vi "Set Toolbar Images.vi"(8 "error in (no error)":errorcluster, 10 "State":T3={"Buttons Displayed"=0, "Button States"=[], "Button Size"=0, "Button Style"=enum."Classic", "Active Button"=0, "Force Regen?"=FALSE, "Tip String Ref"=refnum}) -> (0 "error out":errorcluster, 2 "State Out":T3={"Buttons Displayed"=0, "Button States"=[], "Button Size"=0, "Button Style"=enum."Classic", "Active Button"=0, "Force Regen?"=FALSE, "Tip String Ref"=refnum} caption="State", 3 "Cancelled?":bool)   [LabVIEW 2018, in "Toolbar.xctl"]
doc: "Dialog box to edit the buttons on the toolbar at edit time"
uses:
  Toolbar.xctl
  <vilib>/picture/picture.llb/imagedata.ctl
  Button_Class/Button.lvclass
  Button_Class/Type Defs/Button Status.ctl
  Toolbar State.ctl
  Button_Class/Type Defs/Button Style.ctl
  Button_Class/Type Defs/Button Type.ctl
panel:
  in  "Same Image for all buttons":bool
  out "working Button":refnum<class "Button.lvclass">
  out "Button Images":T1[](array[typedef])
  in  "Button Style":T2 caption="Button Theme"
  in  "Path":path
  in  "Button Sizes":i32
  in  "Current Button":i32
  in  "Buttons Displayed":i32
  in  "Images":enum32{"Off", "Hover", "On", "Disabled"}(tab)
  in  "Paste.Off":bool
  in  "Load.Off":bool
  out "Display.Off":picture
  in  "Paste.Hover":bool
  in  "Load.Hover":bool
  out "Display.Hover":picture
  in  "Paste.On":bool
  in  "Load.On":bool
  out "Display.On":picture
  in  "Paste.Disabled":bool
  in  "Load.Disabled":bool
  out "Display.Disabled":picture
  in  "Type":T4
  in  "Default State":T5
  in  "Cancel":bool
  in  "OK":bool
  # "Toolbar Options"
  # "Button Details"
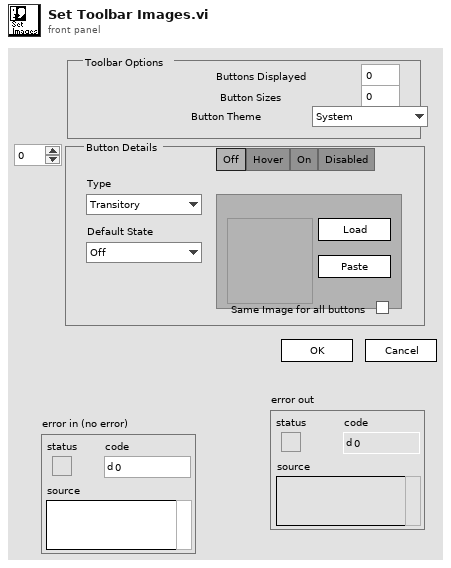
[diagram p1: front panel]
types:
  T1 = typedef "imagedata.ctl" = cluster{"image type":i32, "image depth":i32, "image":u8[], "mask":u8[], "colors":u32[], "Rectangle":cluster{"left":i16, "top":i16, "right":i16, "bottom":i16}}
  T2 = typedef "Button.lvclass/Button Style.ctl" = enum16{"System", "Modern", "Classic", "Rounded", "Silver", "Ni Theme", "Metallic"}
  T3 = typedef "Toolbar.xctl/Toolbar State.ctl" = cluster{"Buttons Displayed":i32, "Button States":refnum<class "Button.lvclass">[], "Button Size":i32, "Button Style":T2, "Active Button":i32, "Force Regen?":bool, "Tip String Ref":refnum<vi>}
  T4 = typedef "Button.lvclass/Button Type.ctl" = enum16{"Transitory", "Latching"}
  T5 = typedef "Button.lvclass/Button Status.ctl" = enum16{"Off", "Hover", "On", "Disabled"}
  T6 = typedef "LVPositionTypeDef.ctl" = cluster{"Left":i32, "Top":i32}
  T7 = typedef "LVBoundsTypeDef.ctl" = cluster{"Width":u32, "Height":u32}
  T8 = enum32{"Page Enabled", "Page Disabled", "Page Disabled & Grayed"}
  T9 = enum32{"existing file", "new file", "new or existing file", "existing dir", "new dir", "new or existing dir", "existing file (use LLBs)", "new file (use LLBs)", "new or existing file (use LLBs)", "new or existing file or directory (use LLBs)", "existing dir (use LLBs)", "new dir (use LLBs)", "new or existing dir (use LLBs)", "existing file or dir", "new file or dir", "new or existing file or dir", "existing file or dir (use LLBs)", "new file or dir (use LLBs)"}
  T10 = typedef "LVRectTypeDef.ctl" = cluster{"left":i16, "top":i16, "right":i16, "bottom":i16}
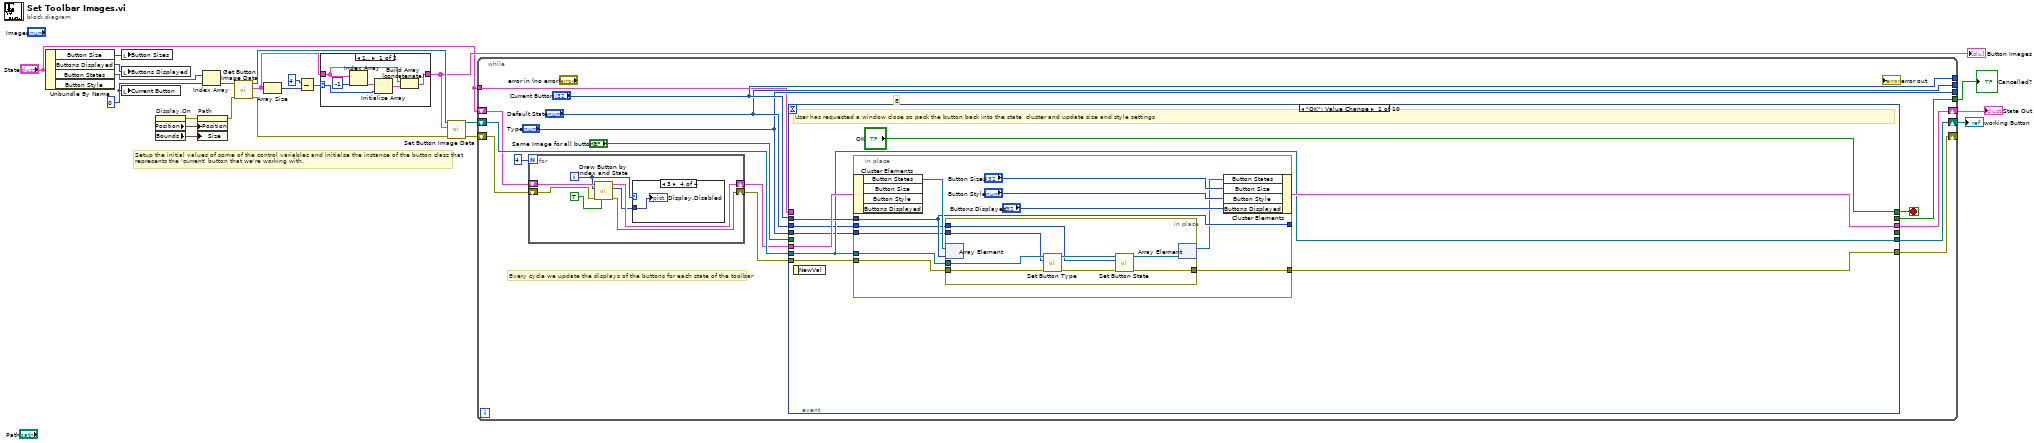
[diagram p0: block diagram]
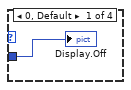
[diagram p3: hidden frame]
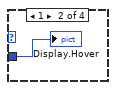
[diagram p4: hidden frame]
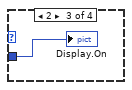
[diagram p5: hidden frame]
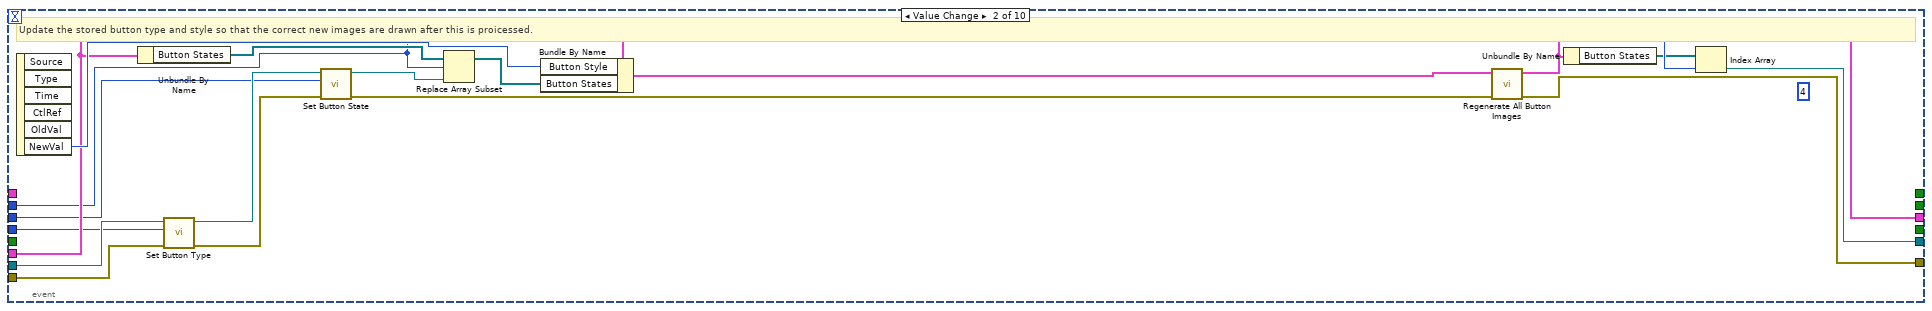
[diagram p6: hidden frame]
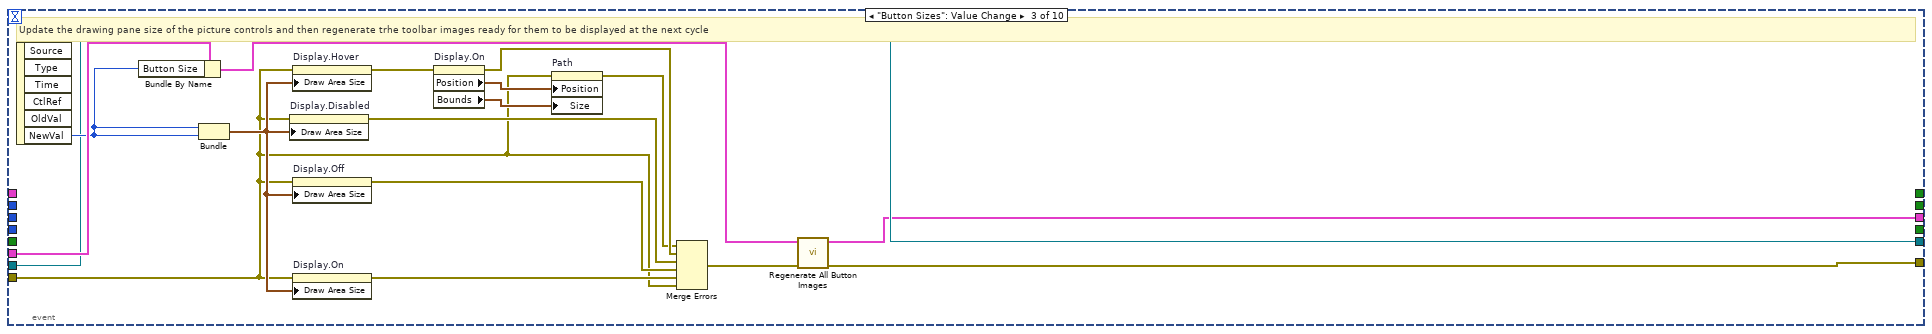
[diagram p7: hidden frame]
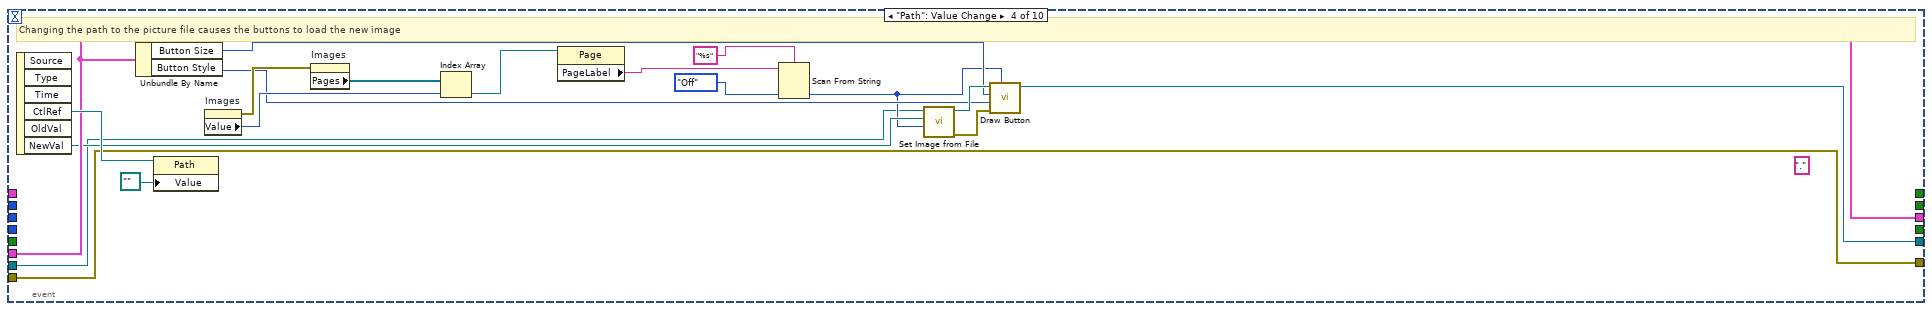
[diagram p8: hidden frame]
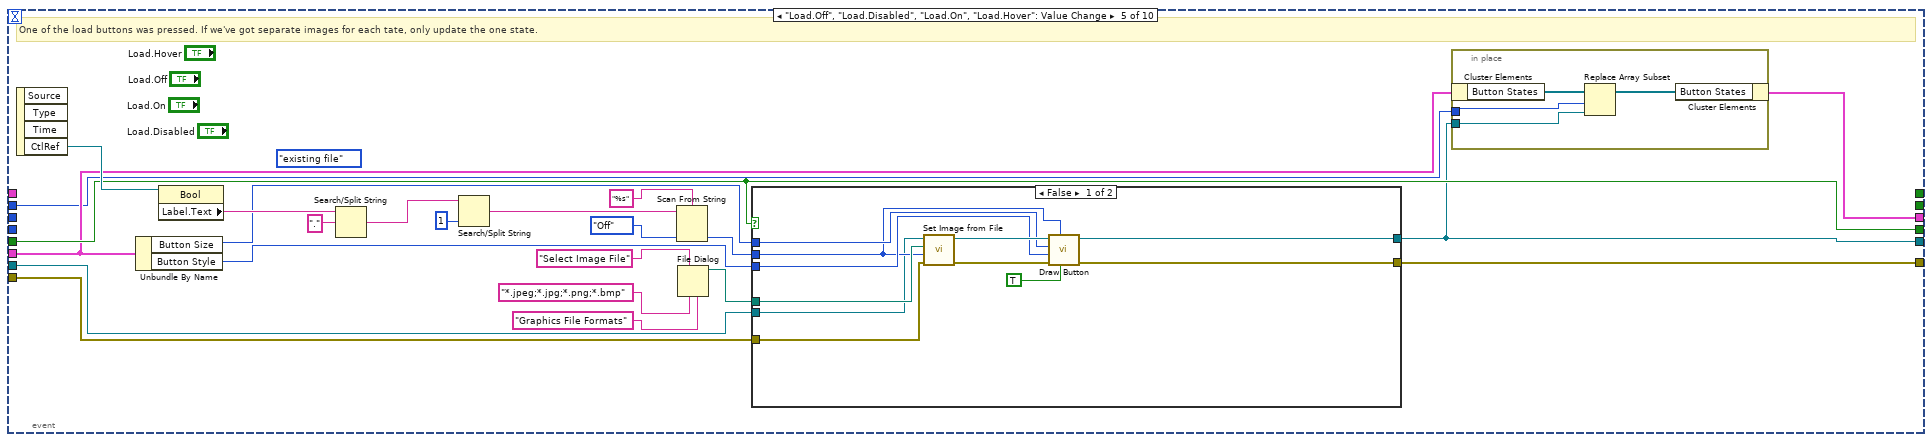
[diagram p9: hidden frame]
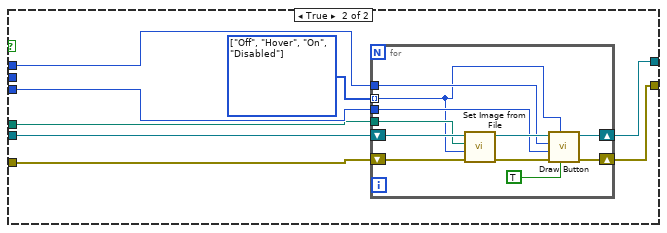
[diagram p10: hidden frame]
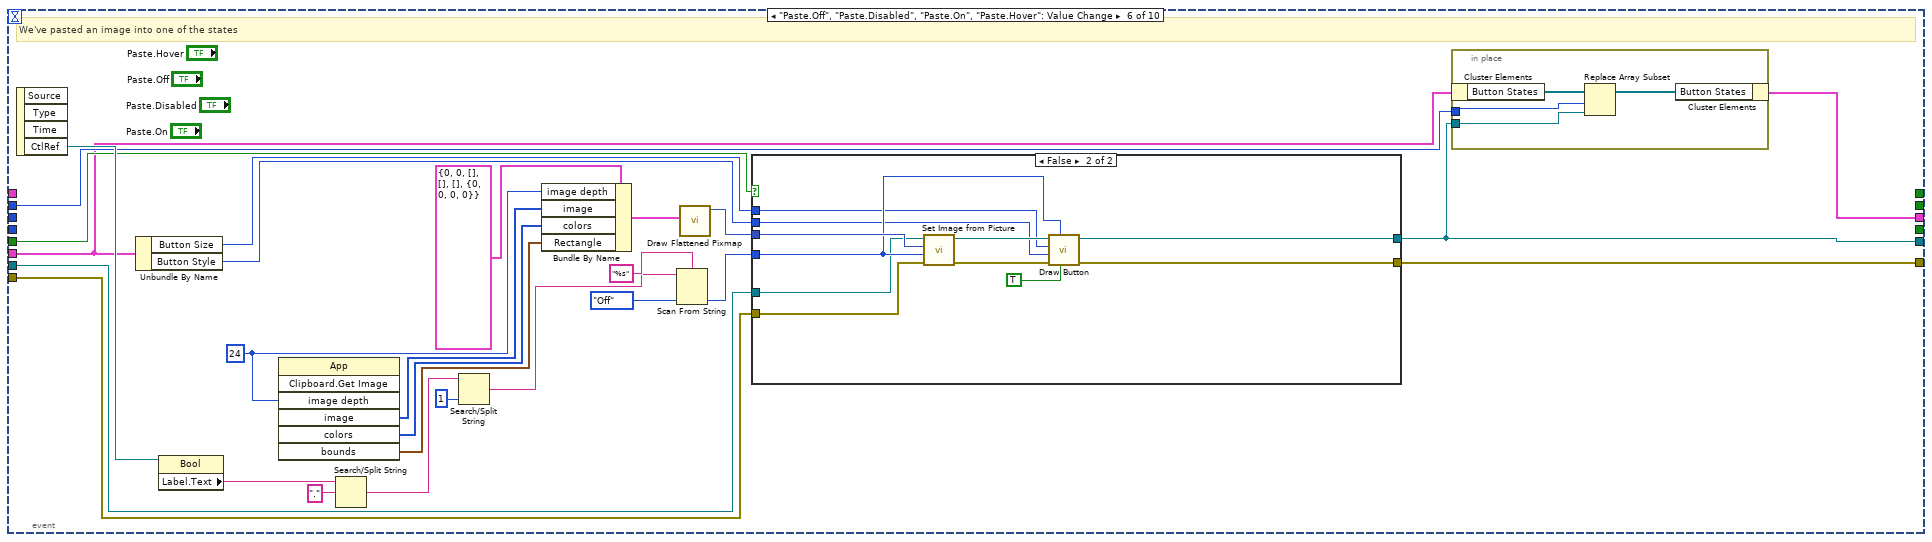
[diagram p11: hidden frame]
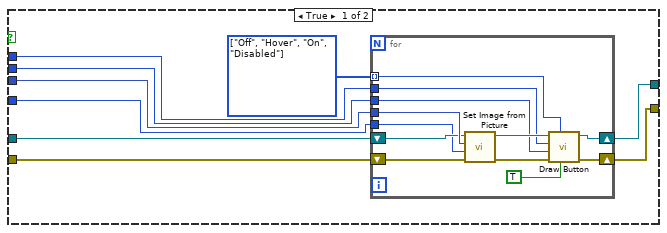
[diagram p12: hidden frame]
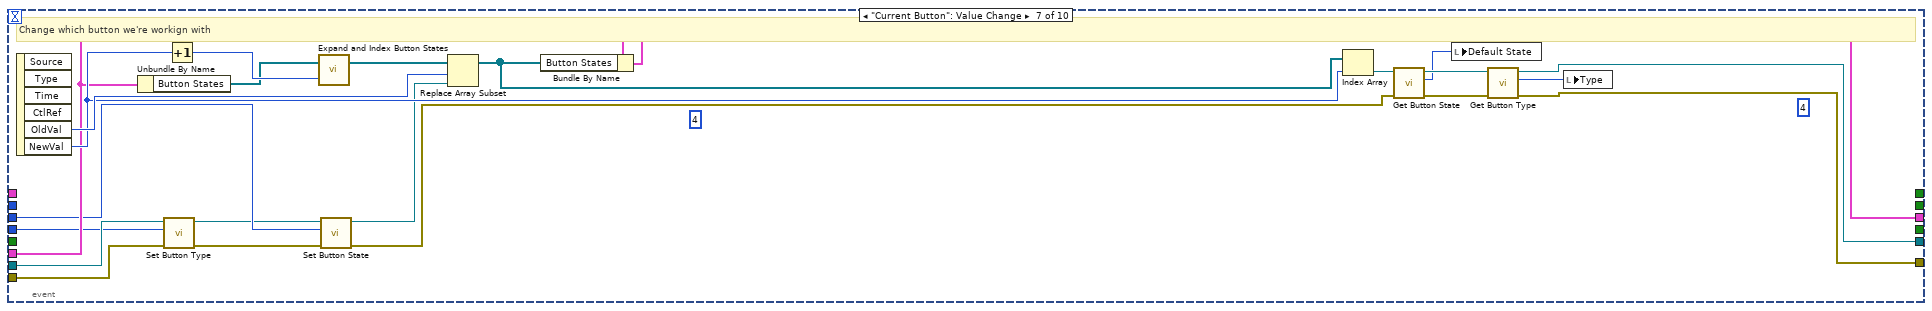
[diagram p13: hidden frame]
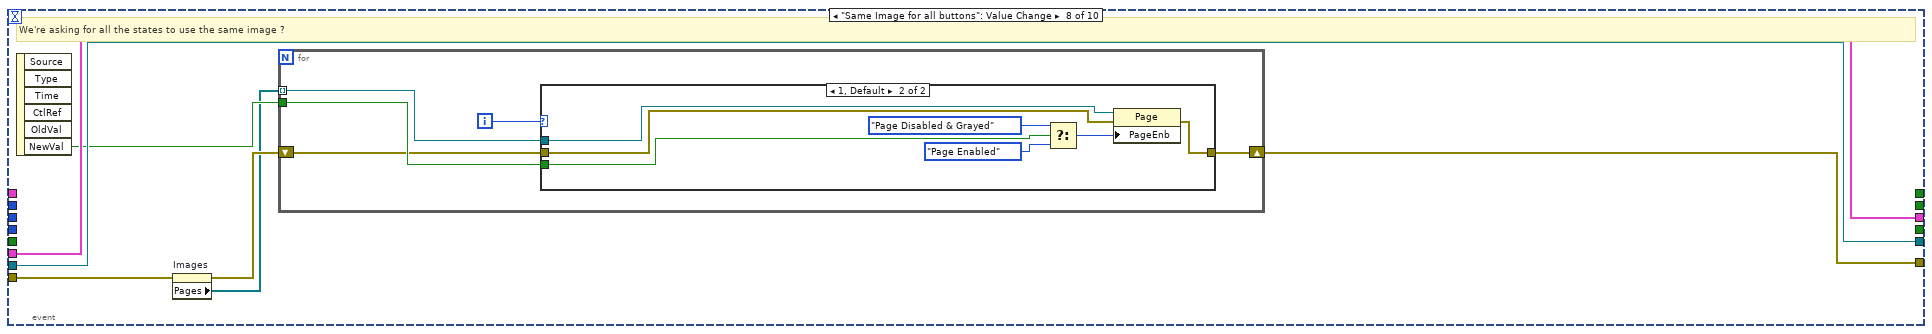
[diagram p14: hidden frame]
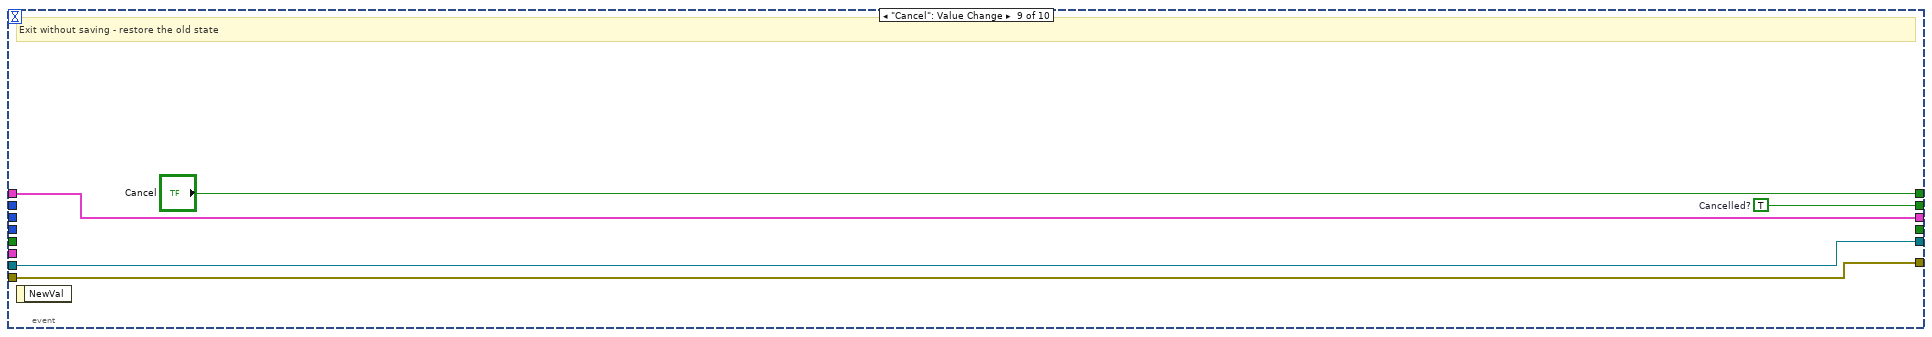
[diagram p16: hidden frame]
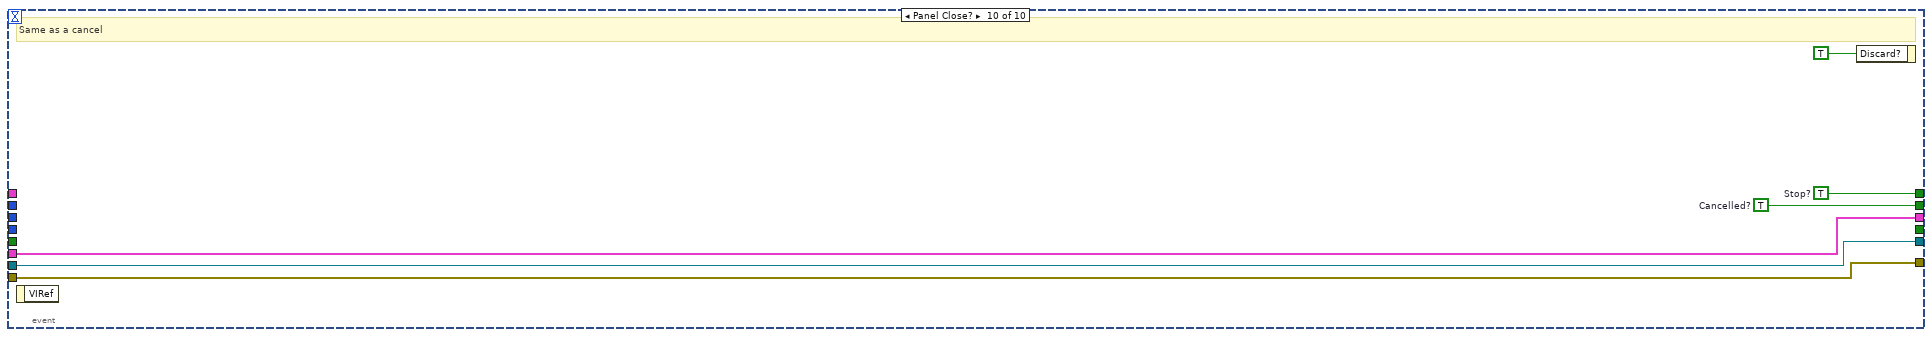
[diagram p17: hidden frame]
diagram:
  w20 = 0 ("Current Button")
  # "Setup the initial values of some of the control variables and initialse the instance of the button class that\nrepresents the 'current' button that we're working with."
  n1 = Unbundle By Name("State") -> ("Button Size"=w19:i32, "Buttons Displayed"=w22:i32, "Button States"=w13:refnum<class "Button.lvclass">[])  [unwired: 1 out]
  n2 = local write "Button Sizes"(w19) -> ()
  n3 = local write "Buttons Displayed"(w22) -> ()
  n4 = local write "Current Button"(w20) -> ()
  n5 = property on="Display.On" class="Pict"() -> (error out=w16:errorcluster, "Position"=w18:T6, "Bounds"=w17:T7)  [unwired: 2 in, 1 out]
  n6 = property on="Path" class="Path"(error in=w16, "Position"=w18, "Size"=w17) -> (error out=w7:errorcluster)  [unwired: 1 in, 1 out]
  n7 = Index Array(array=w13, index=w20) -> (element=w14:refnum<class "Button.lvclass">)
  n8 = call-dynamic "Get Button Image Data.vi"("error in (no error)"=w7, "Button in"=w14) -> ("error out"=w1:errorcluster, "Button Images"=w8:T1[], "Button out"=w15:refnum<class "Button.lvclass">)  [unwired: 7 out]
  n9 = Array Size(array=w8) -> (size(s)=w12:i32)
  n10 = Subtract(x=4 ("Buttons Displayed"), y=w12) -> (x-y=w10:i32)
  n11 = case shown="1.." w10 {
    selector: w10 -> [w27 _]
    tunnel: [w23 w29] -> w9
    tunnel: w8 -> [w25 w29]
    frame 1.. {
      n12 = Index Array(array=w25, index=-1) -> (element=w26:T1)
      n13 = Initialize Array(w26, w27) -> (w24:T1[])
      n14 = Build Array (concatenate)(w25, w24) -> (w23:T1[])
    }
    frame ..0 {
    }
  }
  "Button Images" <- w9
  n15 = call-dynamic "Set Button Image Data.vi"("error in (no error)"=w1, "Button Images"=w9, "Button in"=w15) -> ("error out"=w6:errorcluster, "Button out"=w5:refnum<class "Button.lvclass">)  [unwired: 7 out]
  n16 = while {
    tunnel: [w44] -> w21
    shift-right: [w43] -> w3
    shift-left: "State" -> [w33]
    shift-right: [w42] -> _
    shift-left: w6 -> [w31]
    shift-right: [w40] -> w4
    shift-left: w5 -> [w41]
    tunnel: ["Current Button"] -> _
    tunnel: ["Default State"] -> _
    tunnel: ["Type"] -> _
    tunnel: "State" -> [w34]
    stop <- w45 stop-if-true
    # "Every cycle we update the displays of the buttons for each state of the toolbar"
    # "E"
    n17 = for {
      N: 4 -> [_]
      shift-right: [w51] -> w32
      shift-left: w33 -> [w52]
      shift-right: [w49] -> w30
      shift-left: w31 -> [w50]
      i -> [w47]
      n18 = call "Draw Button by Index and State.vi"("Force redraw ?"=TRUE, "error in (no error)"=w50, "Button State"=w47, "State"=w52) -> ("error out"=w49:errorcluster, "Picture Out"=w46:picture, "State out"=w51:T3)  [unwired: 4 in, 1 out]
      n19 = case shown="3" w47 {
        tunnel: w46 -> [w53 w54 w55 w56]
        frame 0, Default {
          "Display.Off" <- w53
        }
        frame 1 {
          "Display.Hover" <- w54
        }
        frame 2 {
          "Display.On" <- w55
        }
        frame 3 {
          "Display.Disabled" <- w56
        }
      }
    }
    n20 = event shown="[0] \"OK\": Value Change" {
      selector: _ -> [_ _ _ _ _ _ _ _ _ _]
      dyn-events: _ -> [_ _ _ _ _ _ _ _ _ _]
      timeout: _ -> [_ _ _ _ _ _ _ _ _ _]
      tunnel: ["OK" _ _ _ _ _ _ _ "Cancel" w310] -> w45
      tunnel: [_ _ _ _ _ _ _ _ w305 w309] -> w44
      tunnel: w32 -> [w64 w101 w118 w127 w142 w197 w275 w286 _ w308]
      tunnel: [w63 w88 w103 w127 w141 w196 w276 w286 w301 w308] -> w43
      tunnel: w30 -> [w60 w86 w108 w122 w144 w201 w271 w282 w303 w307]
      tunnel: [w59 w87 w105 w122 w143 w200 w258 w281 w303 w307] -> w42
      tunnel: w41 -> [w61 w96 w113 w121 w146 w203 w270 w287 w302 w306]
      tunnel: [w61 w90 w113 w120 w140 w198 w269 w287 w302 w306] -> w40
      tunnel: "Type" -> [w57 w94 _ _ _ _ w267 _ _ _]
      tunnel: "Default State" -> [w58 w93 _ _ _ _ w268 _ _ _]
      tunnel: "Current Button" -> [w62 w92 _ _ w139 w199 _ _ _ _]
      tunnel: [_ _ _ _ w145 _ _ _ _ _] -> _
      tunnel: "Same Image for all buttons" -> [_ _ _ _ w145 w202 _ _ _ _]
      tunnel: w34 -> [_ _ _ _ _ _ _ _ w301 _]
      event "OK": Value Change {
        # "User has requested a window close so pack the button back into the state  cluster and update size and style settings"
        n21 = event-data() -> ()  [unwired: 2 out]
        n22 = in-place {
          in-place-border: [w75] -> _
          in-place-border: w62 -> [w75]
          in-place-border: w61 -> [w74]
          in-place-border: w60 -> [w73]
          in-place-border: [w72] -> w59
          in-place-border: w58 -> [w67]
          in-place-border: w57 -> [w66]
          n23 = in-place-cluster #1(w64) -> ("Button States"=w76:refnum<class "Button.lvclass">[])  [unwired: 3 out]
          n24 = in-place {
            in-place-border: w74 -> [w82]
            in-place-border: w73 -> [w80]
            in-place-border: [w79] -> w72
            in-place-border: w67 -> [w78]
            in-place-border: w66 -> [w77]
            n25 = in-place-array #2(w76, w75) -> ()  [unwired: 1 out]
            n26 = call-dynamic "Set Button Type.vi"("error in (no error)"=w80, "Type"=w77, "Button in"=w82) -> ("error out"=w84:errorcluster, "Button out"=w83:refnum<class "Button.lvclass">)  [unwired: 7 out]
            n27 = call-dynamic "Set Button State.vi"("error in (no error)"=w84, "State"=w78, "Button in"=w83) -> ("error out"=w79:errorcluster, "Button out"=w81:refnum<class "Button.lvclass">)  [unwired: 7 out]
            n28 = in-place-array #2(w81) -> (w68:refnum<class "Button.lvclass">[])  [unwired: 1 out]
          }
          n29 = in-place-cluster #1("Button States"=w68, "Button Size"="Button Sizes", "Button Style"="Button Style", "Buttons Displayed"="Buttons Displayed") -> (w63:T3)
        }
      }
      event Value Change {
        (unwired) 4
        # "Update the stored button type and style so that the correct new images are drawn after this is proicessed."
        n30 = event-data() -> ("NewVal"=w102:T2)  [unwired: 6 out]
        n31 = Unbundle By Name(w101) -> ("Button States"=w97:refnum<class "Button.lvclass">[])
        n32 = call-dynamic "Set Button Type.vi"("error in (no error)"=w86, "Type"=w94, "Button in"=w96) -> ("error out"=w98:errorcluster, "Button out"=w99:refnum<class "Button.lvclass">)  [unwired: 7 out]
        n33 = call-dynamic "Set Button State.vi"("error in (no error)"=w98, "State"=w93, "Button in"=w99) -> ("error out"=w85:errorcluster, "Button out"=w95:refnum<class "Button.lvclass">)  [unwired: 7 out]
        n34 = Replace Array Subset(array=w97, new element=w95, index=w92) -> (w100:refnum<class "Button.lvclass">[])
        n35 = Bundle By Name(cluster=w101, "Button Style"=w102, "Button States"=w100) -> (w89:T3)
        n36 = call "Regenerate All Button Images.vi"("error in (no error)"=w85, "Display State In in"=w89) -> ("error out"=w87:errorcluster, "Display State In out"=w88:T3)  [unwired: 8 in]
        n37 = Unbundle By Name(w88) -> ("Button States"=w91:refnum<class "Button.lvclass">[])
        n38 = Index Array(array=w91, index=w92) -> (element=w90:refnum<class "Button.lvclass">)
      }
      event "Button Sizes": Value Change {
        # "Update the drawing pane size of the picture controls and then regenerate trhe toolbar images ready for them to be displayed at the next cycle"
        n39 = event-data() -> ("NewVal"=w114:i32)  [unwired: 6 out]
        n40 = Bundle By Name(cluster=w118, "Button Size"=w114) -> (w104:T3)
        n41 = Bundle("NewVal"=w114, "NewVal"=w114) -> (w119:cluster{"NewVal":i32, "NewVal":i32})  [unwired: 1 out]
        n42 = property on="Display.Disabled" class="Pict"(error in=w108, "Draw Area Size"=w119) -> (error out=w110:errorcluster)  [unwired: 1 in, 1 out]
        n43 = property on="Display.Hover" class="Pict"(error in=w108, "Draw Area Size"=w119) -> (error out=w115:errorcluster)  [unwired: 1 in, 1 out]
        n44 = property on="Display.Off" class="Pict"(error in=w108, "Draw Area Size"=w119) -> (error out=w111:errorcluster)  [unwired: 1 in, 1 out]
        n45 = property on="Display.On" class="Pict"(error in=w108, "Draw Area Size"=w119) -> (error out=w112:errorcluster)  [unwired: 1 in, 1 out]
        n46 = property on="Display.On" class="Pict"(error in=w115) -> (error out=w109:errorcluster, "Position"=w116:T6, "Bounds"=w117:T7)  [unwired: 1 in, 1 out]
        n47 = property on="Path" class="Path"(error in=w108, "Position"=w116, "Size"=w117) -> (error out=w107:errorcluster)  [unwired: 1 in, 1 out]
        n48 = Merge Errors(w107, w109, w110, w111, w112, w108) -> (w106:errorcluster)
        n49 = call "Regenerate All Button Images.vi"("error in (no error)"=w106, "Display State In in"=w104) -> ("error out"=w105:errorcluster, "Display State In out"=w103:T3)  [unwired: 8 in]
      }
      event "Path": Value Change {
        (unwired) "." ("search string/char (-)")
        # "Changing the path to the picture file causes the buttons to load the new image"
        n50 = event-data() -> ("CtlRef"=w133:refnum<vi>, "NewVal"=w126:path)  [unwired: 5 out]
        n51 = Unbundle By Name(w127) -> ("Button Size"=w125:i32, "Button Style"=w124:T2)
        n52 = property class="Path"(reference=w133, "Value"=path "") -> ()  [unwired: 1 in, 2 out]
        n53 = property on="Images" class="TabCtl (strict)"() -> (error out=w135:errorcluster, "Value"=w136:enum32{"Off", "Hover", "On", "Disabled"})  [unwired: 2 in, 1 out]
        n54 = property on="Images" class="TabCtl (strict)"(error in=w135) -> ("Pages"=w137:refnum<vi>[])  [unwired: 1 in, 2 out]
        n55 = Index Array(array=w137, index=w136) -> (element=w134:refnum<vi>)
        n56 = property class="Page"(reference=w134) -> ("PageLabel"=w130:string)  [unwired: 1 in, 2 out]
        n57 = Scan From String(format string="%s", input string=w130, default 1=Button_Status."Off" ("Button State")) -> (output 1=w123:T5)  [unwired: 2 in, 3 out]
        n58 = call-dynamic "Set Image from File.vi"("State"=w123, "path"=w126, "Button in"=w121) -> ("error out"=w128:errorcluster, "Button out"=w129:refnum<class "Button.lvclass">)  [unwired: 1 in, 6 out]
        n59 = call "Draw Button.vi"("Button State"=w123, "error in (no error)"=w128, "Button Style"=w124, "Button Size"=w125, "Button.lvclass"=w129) -> ("Button.lvclass Out"=w120:refnum<class "Button.lvclass">)  [unwired: 1 in, 5 out]
      }
      event "Load.Off", "Load.Disabled", "Load.On", "Load.Hover": Value Change {
        (unwired) T9."existing file" ("select mode (2)")
        # "One of the load buttons was pressed. If we've got separate images for each tate, only update the one state."
        n60 = event-data() -> ("CtlRef"=w161:refnum<vi>)  [unwired: 4 out]
        n61 = Unbundle By Name(w142) -> ("Button Size"=w149:i32, "Button Style"=w148:T2)
        n62 = property class="Bool"(reference=w161) -> ("Label.Text"=w151:string)  [unwired: 1 in, 2 out]
        n63 = Search/Split String(string=w151, search string/char (-)=".") -> (match + rest of string=w156:string)  [unwired: 3 out]
        n64 = Search/Split String(string=w156, offset (0)=1) -> (match + rest of string=w152:string)  [unwired: 3 out]
        n65 = Scan From String(format string="%s", input string=w152, default 1=Button_Status."Off" ("Button State")) -> (output 1=w147:T5)  [unwired: 2 in, 3 out]
        n66 = File Dialog(4:"Graphics File Formats" ("pattern label"), 6:"*.jpeg;*.jpg;*.png;*.bmp" ("pattern"), 7:"Select Image File" ("prompt")) -> (3:w150:path)  [unwired: 1 in, 6 out]
        n67 = case shown="False" w145 {
          tunnel: w150 -> [w176 w177]
          tunnel: w149 -> [w173 w179]
          tunnel: w148 -> [w172 w180]
          tunnel: w147 -> [w171 _]
          tunnel: w146 -> [w170 w181]
          tunnel: [w169 w182] -> w140
          tunnel: w144 -> [w168 w184]
          tunnel: [w167 w183] -> w143
          frame False {
            n68 = call-dynamic "Set Image from File.vi"("error in (no error)"=w168, "State"=w171, "path"=w176, "Button in"=w170) -> ("error out"=w174:errorcluster, "Button out"=w175:refnum<class "Button.lvclass">)  [unwired: 6 out]
            n69 = call "Draw Button.vi"("Force redraw ?"=TRUE, "Button State"=w171, "error in (no error)"=w174, "Button Style"=w172, "Button Size"=w173, "Button.lvclass"=w175) -> ("error out"=w167:errorcluster, "Button.lvclass Out"=w169:refnum<class "Button.lvclass">)  [unwired: 4 out]
          }
          frame True {
            w178 = T5[] [enum."Off", enum."Hover", enum."On", enum."Disabled"] items=["Off", "Hover", "On", "Disabled"]
            n70 = for {
              shift-right: [w192] -> w183
              shift-left: w184 -> [w193]
              shift-right: [w191] -> w182
              shift-left: w181 -> [w190]
              tunnel: w180 -> [w189]
              tunnel: w179 -> [w188]
              tunnel: w178 -> [w186] mode=indexing
              tunnel: w177 -> [w187]
              n71 = call-dynamic "Set Image from File.vi"("error in (no error)"=w193, "State"=w186, "path"=w187, "Button in"=w190) -> ("error out"=w194:errorcluster, "Button out"=w195:refnum<class "Button.lvclass">)  [unwired: 6 out]
              n72 = call "Draw Button.vi"("Force redraw ?"=TRUE, "Button State"=w186, "error in (no error)"=w194, "Button Style"=w189, "Button Size"=w188, "Button.lvclass"=w195) -> ("error out"=w192:errorcluster, "Button.lvclass Out"=w191:refnum<class "Button.lvclass">)  [unwired: 4 out]
            }
          }
        }
        n73 = in-place {
          in-place-border: w139 -> [w163]
          in-place-border: w140 -> [w162]
          n74 = in-place-cluster #3(w142) -> ("Button States"=w165:refnum<class "Button.lvclass">[])
          n75 = Replace Array Subset(array=w165, new element=w162, index=w163) -> (w164:refnum<class "Button.lvclass">[])
          n76 = in-place-cluster #3("Button States"=w164) -> (w141:T3)
        }
      }
      event "Paste.Off", "Paste.Disabled", "Paste.On", "Paste.Hover": Value Change {
        w217 = 24 ("Image Depth")
        # "We've pasted an image into one of the states"
        n77 = event-data() -> ("CtlRef"=w221:refnum<vi>)  [unwired: 4 out]
        n78 = Unbundle By Name(w197) -> ("Button Size"=w205:i32, "Button Style"=w204:T2)
        n79 = property class="Bool"(reference=w221) -> ("Label.Text"=w220:string)  [unwired: 1 in, 2 out]
        n80 = invoke class="App" method="Clipboard.Get Image"("image depth"=w217) -> ("image"=w216:u8[], "colors"=w215:u32[], "bounds"=w214:T10)  [unwired: 6 in, 4 out]
        n81 = Search/Split String(string=w220, search string/char (-)=".") -> (match + rest of string=w213:string)  [unwired: 3 out]
        n82 = Search/Split String(string=w213, offset (0)=1) -> (match + rest of string=w209:string)  [unwired: 3 out]
        n83 = Bundle By Name(cluster=T1 {"image type"=0, "image depth"=0, "image"=[], "mask"=[], "colors"=[], "Rectangle"={"left"=0, "top"=0, "right"=0, "bottom"=0}} ("image data"), "image depth"=w217, "image"=w216, "colors"=w215, "Rectangle"=w214) -> (w208:T1)
        n84 = Scan From String(format string="%s", input string=w209, default 1=Button_Status."Off" ("Button State")) -> (output 1=w206:T5)  [unwired: 2 in, 3 out]
        n85 = call <vilib>:"Draw Flattened Pixmap.vi"("image data"=w208) -> ("new picture"=w207:picture)  [unwired: 1 in, 7 out]
        n86 = case shown="False" w202 {
          tunnel: w207 -> [w234 w257]
          tunnel: w206 -> [w233 w254]
          tunnel: w205 -> [w232 w253]
          tunnel: w204 -> [w231 w252]
          tunnel: w203 -> [w230 w251]
          tunnel: [w229 w250] -> w198
          tunnel: w201 -> [w227 w249]
          tunnel: [w226 w248] -> w200
          frame True {
            w228 = T5[] [enum."Off", enum."Hover", enum."On", enum."Disabled"] items=["Off", "Hover", "On", "Disabled"]
            n87 = for {
              tunnel: w234 -> [w246]
              tunnel: w233 -> [w239]
              tunnel: w232 -> [w243]
              tunnel: w231 -> [w242]
              tunnel: w228 -> [w238] mode=indexing
              shift-right: [w240] -> w229
              shift-left: w230 -> [w241]
              shift-right: [w236] -> w226
              shift-left: w227 -> [w237]
              n88 = call-dynamic "Set Image from Picture.vi"("error in (no error)"=w237, "State"=w239, "Picture"=w246, "Button in"=w241) -> ("error out"=w245:errorcluster, "Button out"=w244:refnum<class "Button.lvclass">)  [unwired: 1 in, 5 out]
              n89 = call "Draw Button.vi"("Force redraw ?"=TRUE, "Button State"=w238, "error in (no error)"=w245, "Button Style"=w242, "Button Size"=w243, "Button.lvclass"=w244) -> ("error out"=w236:errorcluster, "Button.lvclass Out"=w240:refnum<class "Button.lvclass">)  [unwired: 4 out]
            }
          }
          frame False {
            n90 = call-dynamic "Set Image from Picture.vi"("error in (no error)"=w249, "State"=w254, "Picture"=w257, "Button in"=w251) -> ("error out"=w256:errorcluster, "Button out"=w255:refnum<class "Button.lvclass">)  [unwired: 1 in, 5 out]
            n91 = call "Draw Button.vi"("Force redraw ?"=TRUE, "Button State"=w254, "error in (no error)"=w256, "Button Style"=w252, "Button Size"=w253, "Button.lvclass"=w255) -> ("error out"=w248:errorcluster, "Button.lvclass Out"=w250:refnum<class "Button.lvclass">)  [unwired: 4 out]
          }
        }
        n92 = in-place {
          in-place-border: w199 -> [w223]
          in-place-border: w198 -> [w222]
          n93 = in-place-cluster #4(w197) -> ("Button States"=w225:refnum<class "Button.lvclass">[])
          n94 = Replace Array Subset(array=w225, new element=w222, index=w223) -> (w224:refnum<class "Button.lvclass">[])
          n95 = in-place-cluster #4("Button States"=w224) -> (w196:T3)
        }
      }
      event "Current Button": Value Change {
        (unwired) 4 ("Buttons Displayed")
        (unwired) 4
        # "Change which button we're workign with"
        n96 = event-data() -> ("OldVal"=w279:i32, "NewVal"=w278:i32)  [unwired: 5 out]
        n97 = Unbundle By Name(w275) -> ("Button States"=w273:refnum<class "Button.lvclass">[])
        n98 = call-dynamic "Set Button Type.vi"("error in (no error)"=w271, "Type"=w267, "Button in"=w270) -> ("error out"=w265:errorcluster, "Button out"=w266:refnum<class "Button.lvclass">)  [unwired: 7 out]
        n99 = Increment(x=w278) -> (x+1=w277:i32)
        n100 = call "Expand and Index Button States.vi"("Button Index"=w277, "Button States"=w273) -> ("Button States Out"=w274:refnum<class "Button.lvclass">[])  [unwired: 1 out]
        n101 = call-dynamic "Set Button State.vi"("error in (no error)"=w265, "State"=w268, "Button in"=w266) -> ("error out"=w272:errorcluster, "Button out"=w264:refnum<class "Button.lvclass">)  [unwired: 7 out]
        n102 = Replace Array Subset(array=w274, new element=w264, index=w279) -> (w280:refnum<class "Button.lvclass">[])
        n103 = Bundle By Name(cluster=w275, "Button States"=w280) -> (w276:T3)
        n104 = Index Array(array=w280, index=w278) -> (element=w263:refnum<class "Button.lvclass">)
        n105 = call-dynamic "Get Button State.vi"("error in (no error)"=w272, "Button in"=w263) -> ("error out"=w259:errorcluster, "State"=w261:T5, "Button out"=w262:refnum<class "Button.lvclass">)  [unwired: 7 out]
        n106 = local write "Default State"(w261) -> ()
        n107 = call-dynamic "Get Button Type.vi"("error in (no error)"=w259, "Button in"=w262) -> ("error out"=w258:errorcluster, "Type"=w260:T4, "Button out"=w269:refnum<class "Button.lvclass">)  [unwired: 7 out]
        n108 = local write "Type"(w260) -> ()
      }
      event "Same Image for all buttons": Value Change {
        # "We're asking for all the states to use the same image ?"
        n109 = event-data() -> ("NewVal"=w284:bool)  [unwired: 6 out]
        n110 = property on="Images" class="TabCtl (strict)"(error in=w282) -> (error out=w285:errorcluster, "Pages"=w283:refnum<vi>[])  [unwired: 1 in, 1 out]
        n111 = for {
          shift-right: [w288] -> w281
          shift-left: w285 -> [w289]
          tunnel: w284 -> [w291]
          tunnel: w283 -> [w290] mode=indexing
          i -> [w292]
          n112 = case shown="1, Default" w292 {
            tunnel: w291 -> [_ w295]
            tunnel: w290 -> [_ w300]
            tunnel: w289 -> [w293 w299]
            tunnel: [w293 w298] -> w288
            frame 0 {
            }
            frame 1, Default {
              n113 = Select(t=T8."Page Disabled & Grayed" ("Page Enabled State"), s=w295, f=T8."Page Enabled" ("Page Enabled State")) -> (s? t:f=w294:T8)
              n114 = property class="Page"(reference=w300, error in=w299, "PageEnb"=w294) -> (error out=w298:errorcluster)  [unwired: 1 out]
            }
          }
        }
      }
      event "Cancel": Value Change {
        w305 = TRUE  # Cancelled?
        # "Exit without saving - restore the old state"
        n115 = event-data() -> ()  [unwired: 2 out]
      }
      event Panel Close? {
        w309 = TRUE  # Cancelled?
        w310 = TRUE  # Stop?
        # "Same as a cancel"
        n116 = event-data() -> ()  [unwired: 2 out]
        n117 = event-data("Discard?"=TRUE) -> ()  [unwired: 1 in, 1 out]
      }
    }
  }
  "Cancelled?" <- w21
  "State Out" <- w3
  "working Button" <- w4
